vi "Test Assert Not Equal Type.vi"(8 "error in (no error)":errorcluster) -> (0 "error out":errorcluster)   [LabVIEW 2009]
uses:
  classes/Assert/Assert.lvclass
  classes/Test Suite/Test Suite.lvclass
  classes/Test/Test.lvclass
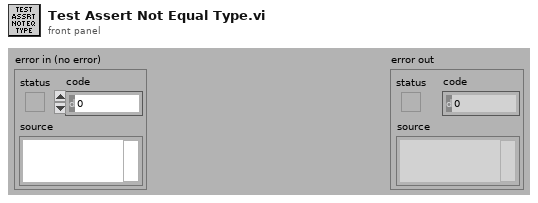
[diagram p1: front panel]
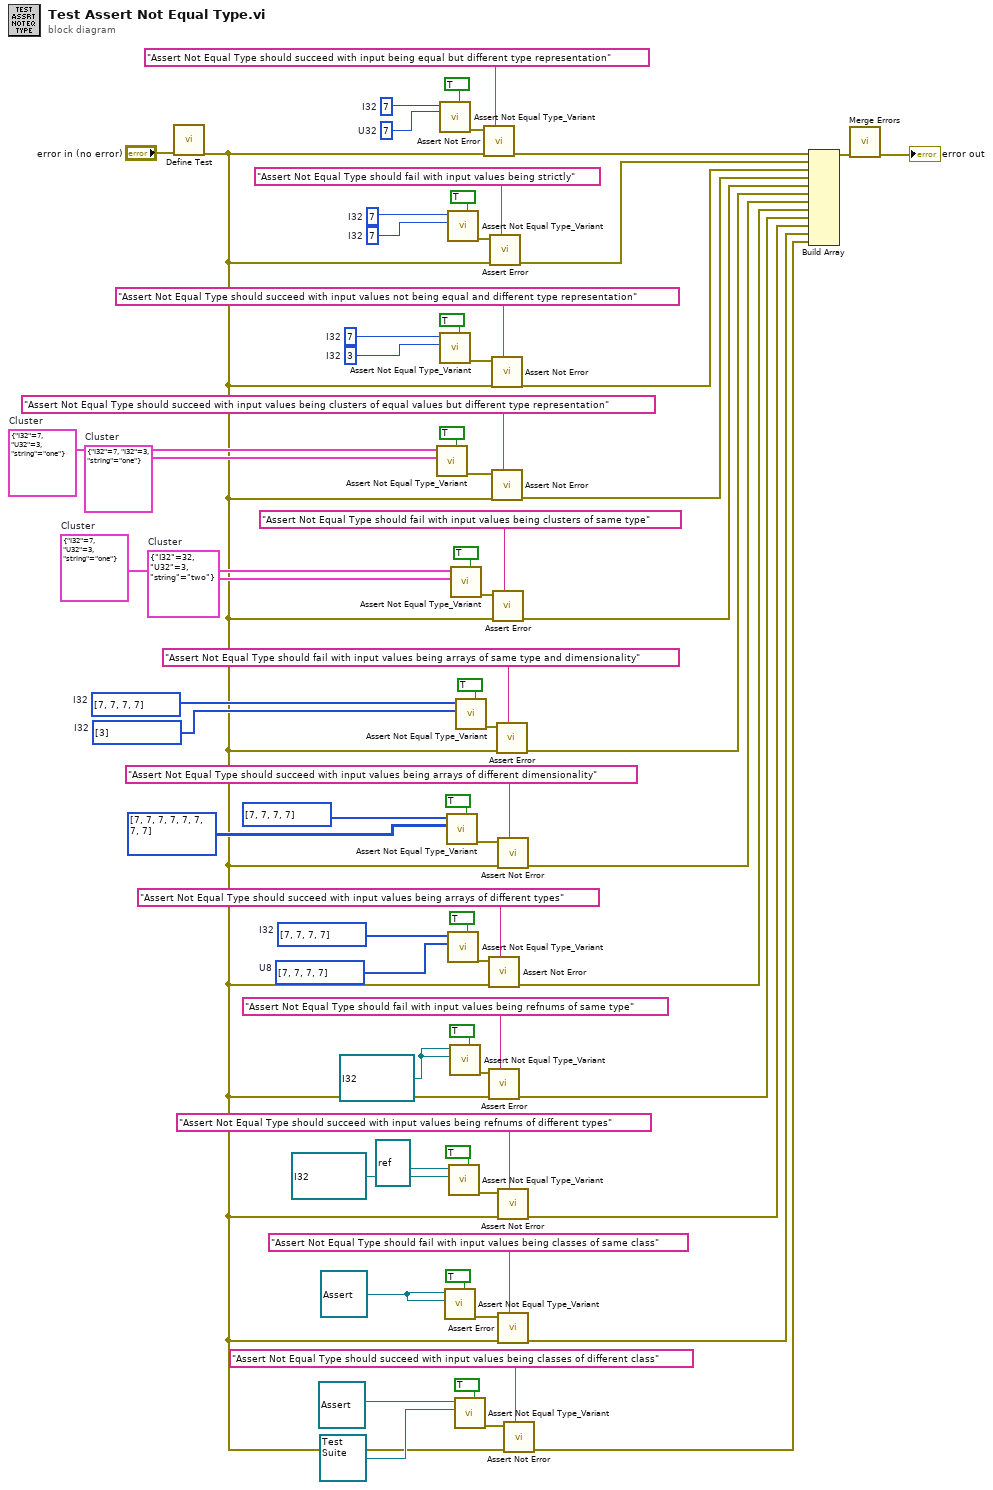
[diagram p0: block diagram]
diagram:
  w3 = refnum<class "Assert.lvclass"> refnum ("Caraya.lvlib:Assert.lvclass")
  w32 = u32 7  # U32
  w16 = refnum<queue> refnum ("queue out")
  w34 = u8[] [7, 7, 7, 7]  # U8
  w35 = i32[] [7, 7, 7, 7]  # I32
  w20 = i32[] [3]  # I32
  w21 = i32[] [7, 7, 7, 7]  # I32
  w28 = cluster{"I32":i32, "I32":i32, "string":string} {"I32"=7, "I32"=3, "string"="one"}  # Cluster
  w29 = cluster{"I32":i32, "U32":u32, "string":string} {"I32"=7, "U32"=3, "string"="one"}  # Cluster
  w26 = cluster{"I32":i32, "U32":u32, "string":string} {"I32"=32, "U32"=3, "string"="two"}  # Cluster
  w27 = cluster{"I32":i32, "U32":u32, "string":string} {"I32"=7, "U32"=3, "string"="one"}  # Cluster
  w53 = 7  # I32
  w54 = 7  # I32
  w59 = 7  # I32
  w49 = u32 3  # I32
  w50 = 7  # I32
  n1 = call "Define Test.vi"("error in (no error)"="error in (no error)") -> ("error out"=w4:errorcluster)  [unwired: 10 in]
  n2 = call "Assert Not Equal Type_Variant.vi"("Assert Only? (F)"=TRUE, "Y"=w28, "X"=w29) -> ("error out"=w48:errorcluster)  [unwired: 8 in]
  n3 = call "Assert Not Equal Type_Variant.vi"("Assert Only? (F)"=TRUE, "Y"=w32, "X"=w59) -> ("error out"=w57:errorcluster)  [unwired: 8 in]
  n4 = call "Assert Not Equal Type_Variant.vi"("Assert Only? (F)"=TRUE, "Y"=w49, "X"=w50) -> ("error out"=w52:errorcluster)  [unwired: 8 in]
  n5 = call "Assert Not Equal Type_Variant.vi"("Assert Only? (F)"=TRUE, "Y"=w3, "X"=w3) -> ("error out"=w7:errorcluster)  [unwired: 8 in]
  n6 = call "Assert Not Equal Type_Variant.vi"("Assert Only? (F)"=TRUE, "Y"=i32[][] [[7, 7, 7, 7], [7, 7, 7, 7]], "X"=i32[] [7, 7, 7, 7]) -> ("error out"=w42:errorcluster)  [unwired: 8 in]
  n7 = call "Assert Not Equal Type_Variant.vi"("Assert Only? (F)"=TRUE, "Y"=w53, "X"=w54) -> ("error out"=w56:errorcluster)  [unwired: 8 in]
  n8 = call "Assert Not Equal Type_Variant.vi"("Assert Only? (F)"=TRUE, "Y"=w34, "X"=w35) -> ("error out"=w17:errorcluster)  [unwired: 8 in]
  n9 = call "Assert Not Equal Type_Variant.vi"("Assert Only? (F)"=TRUE, "Y"=refnum<queue> refnum ("queue out"), "X"=refnum<vi> refnum ("This VI")) -> ("error out"=w39:errorcluster)  [unwired: 8 in]
  n10 = call "Assert Not Equal Type_Variant.vi"("Assert Only? (F)"=TRUE, "Y"=w16, "X"=w16) -> ("error out"=w40:errorcluster)  [unwired: 8 in]
  n11 = call "Assert Not Equal Type_Variant.vi"("Assert Only? (F)"=TRUE, "Y"=w26, "X"=w27) -> ("error out"=w46:errorcluster)  [unwired: 8 in]
  n12 = call "Assert Not Equal Type_Variant.vi"("Assert Only? (F)"=TRUE, "Y"=refnum<class "Test Suite.lvclass"> refnum ("Caraya.lvlib:Test Suite.lvclass"), "X"=refnum<class "Assert.lvclass"> refnum ("Caraya.lvlib:Assert.lvclass")) -> ("error out"=w6:errorcluster)  [unwired: 8 in]
  n13 = call "Assert Not Equal Type_Variant.vi"("Assert Only? (F)"=TRUE, "Y"=w20, "X"=w21) -> ("error out"=w44:errorcluster)  [unwired: 8 in]
  n14 = call "Assert Not Error.vi"("Label"="Assert Not Equal Type should succeed with input being equal but different type representation", "error in (no error)"=w4, "Not Error?"=w57) -> ("error out"=w70:errorcluster)  [unwired: 8 in]
  n15 = call "Assert Not Error.vi"("Label"="Assert Not Equal Type should succeed with input values being arrays of different types", "error in (no error)"=w4, "Not Error?"=w17) -> ("error out"=w19:errorcluster)  [unwired: 8 in]
  n16 = call "Assert Error.vi"("Label"="Assert Not Equal Type should fail with input values being refnums of same type", "error in (no error)"=w4, "Error?"=w40) -> ("error out"=w61:errorcluster)  [unwired: 8 in]
  n17 = call "Assert Error.vi"("Label"="Assert Not Equal Type should fail with input values being strictly", "error in (no error)"=w4, "Error?"=w56) -> ("error out"=w69:errorcluster)  [unwired: 8 in]
  n18 = call "Assert Not Error.vi"("Label"="Assert Not Equal Type should succeed with input values not being equal and different type representation", "error in (no error)"=w4, "Not Error?"=w52) -> ("error out"=w67:errorcluster)  [unwired: 8 in]
  n19 = call "Assert Not Error.vi"("Label"="Assert Not Equal Type should succeed with input values being clusters of equal values but different type representation", "error in (no error)"=w4, "Not Error?"=w48) -> ("error out"=w65:errorcluster)  [unwired: 8 in]
  n20 = call "Assert Error.vi"("Label"="Assert Not Equal Type should fail with input values being clusters of same type", "error in (no error)"=w4, "Error?"=w46) -> ("error out"=w64:errorcluster)  [unwired: 8 in]
  n21 = call "Assert Error.vi"("Label"="Assert Not Equal Type should fail with input values being arrays of same type and dimensionality", "error in (no error)"=w4, "Error?"=w44) -> ("error out"=w63:errorcluster)  [unwired: 8 in]
  n22 = call "Assert Not Error.vi"("Label"="Assert Not Equal Type should succeed with input values being arrays of different dimensionality", "error in (no error)"=w4, "Not Error?"=w42) -> ("error out"=w62:errorcluster)  [unwired: 8 in]
  n23 = call "Assert Not Error.vi"("Label"="Assert Not Equal Type should succeed with input values being refnums of different types", "error in (no error)"=w4, "Not Error?"=w39) -> ("error out"=w60:errorcluster)  [unwired: 8 in]
  n24 = call "Assert Error.vi"("Label"="Assert Not Equal Type should fail with input values being classes of same class", "error in (no error)"=w4, "Error?"=w7) -> ("error out"=w2:errorcluster)  [unwired: 8 in]
  n25 = call "Assert Not Error.vi"("Label"="Assert Not Equal Type should succeed with input values being classes of different class", "error in (no error)"=w4, "Not Error?"=w6) -> ("error out"=w1:errorcluster)  [unwired: 8 in]
  n26 = Build Array(w70, w69, w67, w65, w64, w63, w62, w19, w61, w60, w2, w1) -> (w68:errorcluster[])
  n27 = call <vilib>:"Merge Errors.vi"("error array in"=w68) -> ("error out"=→"error out":errorcluster)  [unwired: 6 in]
